vi "Example 04 - Global Variables.vi"() -> ()   [LabVIEW 2020]
uses:
  Lua for LabVIEW/Lua/Lua.lvclass
panel:
  in  "x":dbl=-2.5 format="%#_13g"
  in  "y":dbl=4.6 format="%#_13g"
  out "error out":errorcluster
  out "z":dbl
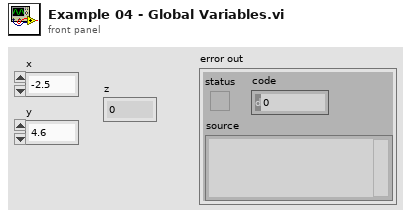
[diagram p1: front panel]
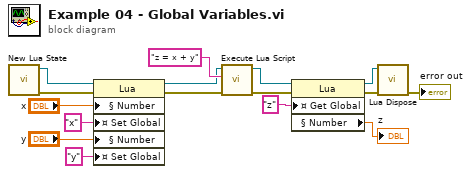
[diagram p0: block diagram]
diagram:
  n1 = call "New Lua State.vi"() -> ("error out"=w16:errorcluster, "Lua out"=w10:refnum<data-value>)  [unwired: 10 in]
  n2 = property class="Lua"(reference=w10, error in=w16, "§ Number"="x", "¤ Set Global"="x" ("(State) Get Global"), "§ Number"="y", "¤ Set Global"="y" ("(State) Get Global")) -> (reference out=w1:refnum<data-value>, error out=w4:errorcluster)
  n3 = call "Execute Lua Script.vi"("error in (no error)"=w4, "lua script"="z = x + y", "Lua in"=w1) -> ("error out"=w5:errorcluster, "Lua out"=w6:refnum<data-value>)  [unwired: 7 in]
  n4 = property class="Lua"(reference=w6, error in=w5, "¤ Get Global"="z") -> (reference out=w13:refnum<data-value>, error out=w12:errorcluster, "§ Number"=→"z":dbl)
  n5 = call "Lua Dispose.vi"("error in (no error)"=w12, "Disposable in"=w13) -> ("error out"=→"error out":errorcluster)  [unwired: 9 in]
